vi "OutputBallHandling.vi"   [LabVIEW 2023]
doc: "This VI sends commands to the arm subsystem."
uses:
  GlobalBallHandling.vi
  GRNF_CTREMotor.vi
types:
  T1 = enum16{"No Changed Output", "New Normal Output", "New Testing Output"}
  T2 = typedef "WPI_MotorControlDeviceRef.ctl" = cluster{"DeviceStatus":errorcluster, "Type":T3, "PWM":cluster{"PWM Channel":T4, "DeadBand":T5}, "CAN":cluster{"Device Number":u8, "SetOutput VI Ref":variant, "GetOutput VI Ref":variant, "Enable VI Ref":variant, "Disable VI Ref":variant, "Data":variant}, "Invert":bool, "DIO PWM":cluster{"PWM \"Enable\" Channel":T4, "DIOChannel":T6, "PWM Rate":dbl}}
  T3 = typedef "WPI_MotorControlType.ctl" = enum16{"PWM", "CAN", "DIO PWM"}
  T4 = typedef "FPGA_DIOPWMChannel.ctl" = enum8{"PWM 0", "PWM 1", "PWM 2", "PWM 3", "PWM 4", "PWM 5", "PWM 6", "PWM 7", "PWM 8", "PWM 9", "PWM MXP 0", "PWM MXP 1", "PWM MXP 2", "PWM MXP 3", "PWM MXP 4", "PWM MXP 5", "PWM MXP 6", "PWM MXP 7", "PWM MXP 8", "PWM MXP 9", "Invalid"}
  T5 = typedef "WPI_PWMDeadband.ctl" = cluster{"Name":string, "maxPositivePwm":i32, "minPositivePwm":i32, "centerPwm":i32, "maxNegativePwm":i32, "minNegativePwm":i32, "angularRange":u16}
  T6 = typedef "FPGA_DIOChannel.ctl" = enum8{"DIO 0", "DIO 1", "DIO 2", "DIO 3", "DIO 4", "DIO 5", "DIO 6", "DIO 7", "DIO 8", "DIO 9", "DIO MXP 0", "DIO MXP 1", "DIO MXP 2", "DIO MXP 3", "DIO MXP 4", "DIO MXP 5", "DIO MXP 6", "DIO MXP 7", "DIO MXP 8", "DIO MXP 9", "DIO MXP 10", "DIO MXP 11", "DIO MXP 12", "DIO MXP 13", "DIO MXP 14", "DIO MXP 15", "SPI Port CS1", "SPI Port CS2", "SPI Port CS3", "SPI Port MISO", "SPI Port MOSI", "Invalid"}
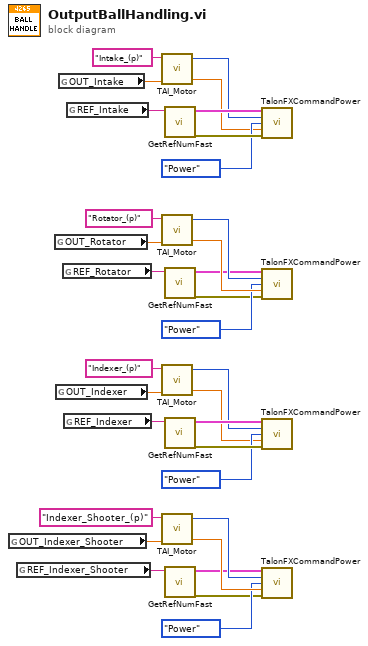
[diagram p0: block diagram]
diagram:
  n1 = global read "GlobalBallHandling.vi" "OUT_Indexer_Shooter"() -> (w8:dbl)
  n2 = global read "GlobalBallHandling.vi" "REF_Indexer_Shooter"() -> (w7:string)
  n3 = global read "GlobalBallHandling.vi" "OUT_Rotator"() -> (w24:dbl)
  n4 = global read "GlobalBallHandling.vi" "OUT_Indexer"() -> (w9:dbl)
  n5 = global read "GlobalBallHandling.vi" "OUT_Intake"() -> (w25:dbl)
  n6 = global read "GlobalBallHandling.vi" "REF_Rotator"() -> (w23:string)
  n7 = global read "GlobalBallHandling.vi" "REF_Indexer"() -> (w10:string)
  n8 = global read "GlobalBallHandling.vi" "REF_Intake"() -> (w26:string)
  n9 = call "TAI_Motor.vi"("Normal Output"=w25, "Actuator Name"="Intake_(p)") -> ("Interlocked Output"=w27:dbl, "Testing Mode"=w28:T1)  [unwired: 3 in]
  n10 = call "TAI_Motor.vi"("Normal Output"=w24, "Actuator Name"="Rotator_(p)") -> ("Interlocked Output"=w22:dbl, "Testing Mode"=w21:T1)  [unwired: 3 in]
  n11 = call "TAI_Motor.vi"("Normal Output"=w9, "Actuator Name"="Indexer_(p)") -> ("Interlocked Output"=w11:dbl, "Testing Mode"=w12:T1)  [unwired: 3 in]
  n12 = call "TAI_Motor.vi"("Normal Output"=w8, "Actuator Name"="Indexer_Shooter_(p)") -> ("Interlocked Output"=w6:dbl, "Testing Mode"=w5:T1)  [unwired: 3 in]
  n13 = call-poly "GetRefNumFast.vi"("RefNum Name"=w26) -> ("Error"=w30:errorcluster, "Device Reference"=w31:T2)  [unwired: 5 in]
  n14 = call-poly "GetRefNumFast.vi"("RefNum Name"=w23) -> ("Error"=w19:errorcluster, "Device Reference"=w18:T2)  [unwired: 5 in]
  n15 = call-poly "GetRefNumFast.vi"("RefNum Name"=w10) -> ("Error"=w14:errorcluster, "Device Reference"=w15:T2)  [unwired: 5 in]
  n16 = call-poly "GetRefNumFast.vi"("RefNum Name"=w7) -> ("Error"=w3:errorcluster, "Device Reference"=w2:T2)  [unwired: 5 in]
  n17 = call "TalonFXCommandPower.vi"("Device Reference (in)"=w31, "Output Mode"=w28, "Control Mode"=enum16{"Safety", "Power"}."Power", "Power or Testing Power"=w27, "Error (in)"=w30) -> ()  [unwired: 11 in]
  n18 = call "TalonFXCommandPower.vi"("Device Reference (in)"=w18, "Output Mode"=w21, "Control Mode"=enum16{"Safety", "Power"}."Power", "Power or Testing Power"=w22, "Error (in)"=w19) -> ()  [unwired: 11 in]
  n19 = call "TalonFXCommandPower.vi"("Device Reference (in)"=w15, "Output Mode"=w12, "Control Mode"=enum16{"Safety", "Power"}."Power", "Power or Testing Power"=w11, "Error (in)"=w14) -> ()  [unwired: 11 in]
  n20 = call "TalonFXCommandPower.vi"("Device Reference (in)"=w2, "Output Mode"=w5, "Control Mode"=enum16{"Safety", "Power"}."Power", "Power or Testing Power"=w6, "Error (in)"=w3) -> ()  [unwired: 11 in]
